vi "Version_4.9_8_on-chip_valves_for25ulSyringe_withModfied_Plunging.vi"() -> ()   [LabVIEW 2020]
uses:
  C:/Users/Admin/Desktop/MicroPurification/Developer/MainLabViewProject_V2.0/Thorlabs/Thorlabs.MotionControl.Controls.dll
  MainLabViewProject_V2.0/Thorlabs/Thorlabs.MotionControl.Controls.dll
  C:/Users/Admin/Desktop/MicroPurification/Developer/MainLabViewProject_V2.0/Thorlabs/Thorlabs.MotionControl.KCube.InertialMotorCLI.dll
  MainLabViewProject_V2.0/Thorlabs/Thorlabs.MotionControl.KCube.InertialMotorCLI.dll
  <vilib>/Instr/_visa.llb/VISA Configure Serial Port (Instr).vi
  <vilib>/Waveform/WDTOps.llb/WDT Append Waveforms DBL.vi
  <vilib>/Fluigent/Fluigent SDK/sourceCode/fgt_SDK.lvlib
panel:
  in  "Set - Blotting Time":bool
  in  "Set - Blotting Angle":bool
  in  "Automated Blotting \nand Plunging":bool=TRUE
  in  "Blotting Time":dbl=1000.0
  in  "Blotting Angle":dbl=10.0
  in  "Amount of \nGrid Shift \nfor Blotting (um)":i32
  out "Ethane Temperature":dbl
  out "RH (%)":dbl
  out "Valve Closing \nPressure Measured":sgl
  out "Suction pressure \nmeasured":sgl
  in  "Divert Elution Buffer\ninto Column-1":bool
  in  "Discard volume \npriot to elution":dbl=1.0
  in  "Buffer-B Dispense\nFlow Rate for Elution \ntubing pre-wash":dbl=2.0
  in  "Buffer-B Volume \nfor elution tubing \npre-wash":dbl=20.0
  in  "External Valve \nOpen":bool
  in  "N-B1":i32=4
  in  "Valve V10 Open":bool=TRUE
  in  "Valve V9 Open":bool=TRUE
  in  "Valve V8 Open":bool=TRUE
  in  "Capillary purge \nvolume after every\ngrid plunging":dbl=0.05
  in  "Automatic purging \nof capillary after \ngrid deposition":bool=TRUE
  in  "No. of \ncleaning cycles":i32=4
  in  "Pause Elution\nValue":dbl
  in  "Re-SEC":bool
  in  "Buffer-C2 Dispense \nFlow Rate for Washing \nPrior to re-introducing Sample":dbl=2.0
  in  "Buffer-C2 \nWash Volume\nPrior to re-introducing \nSample":dbl=20.0
  in  "Wash column-2 Prior \nto re-introducing \nsample":bool=TRUE
  in  "Valve V7 Open":bool=TRUE
  in  "Valve V6 Open":bool=TRUE
  in  "Valve V5 Open":bool=TRUE
  in  "Fluigent\nLink S/N":u16=10704
  in  "Move Grid \nDown Faster":dbl
  in  "Move Grid \nUp Faster":dbl
  in  "Affinity Elution \nGraph Min CutOff":dbl=1.0
  out "Affinity Elution \nis Approaching":bool
  out "Elution of Column-2":bool
  in  "Port for \nC2-Elution":string="5"
  out "Elution of Column-1":bool
  in  "Port for \nB-Elution":string="7"
  in  "f":dbl
  out "Washing Column-2":bool
  out "Washing Column-1":bool
  in  "Port for \nA2-Wash":string="4"
  out "Sample pumping \ninto Column-1":bool
  out "Equilibriating \nColumn-2":bool
  out "Equilibriating \nColumn-1":bool
  in  "V-S":dbl=10.0
  in  "Port for \nSample":string="3"
  in  "N-S":i32=1
  in  "External Valve \nCLOSED":string="2"
  in  "External Valve \nOPEN":string="1"
  in  "Port for \nC1-Equilibriation":string="5"
  in  "Port for \nA1-Equilibriation":string="4"
  in  "Port-<n> to be \nCleaned (4-9)":i32(ring) items=["4", "5", "6", "7", "8", "9"]
  in  "Clean the \nBuffer-C2 tubing":bool
  in  "Clean the \nBuffer-B tubing":bool=TRUE
  in  "Signal":bool
  out "Net Elution \nVolume":dbl
  out "Pause Elution":bool
  in  "Apparent Volume\nof Syringe":dbl=20.0
  in  "N-C1":i32=4
  in  "N-A1":i32=4
  in  "On-Chip Valve \nClosing\nPressure (mbar)":dbl=1200.0
  in  "Wait time for\ntranslation":u32=100
  out "Suction pressure \nfor grid deposition":sgl
  in  "Suction Pressure\nfor EM-grid \nDeposition (mbar)":sgl
  out "Amplified Signal with Fluid Volume for Affinity Elution":cluster{"Array":dbl[], "Array":dbl[]}(graph)
  out "Affinity Elution On":bool
  out "Amplified Signal with Fluid Volume Near Affinity Elution":cluster{"Array":dbl[], "Array":dbl[]}(graph)
  in  "Valve V4 Open":bool=TRUE
  out "Affinity On":bool
  out "Amplified Signal with Fluid Volume for SEC":cluster{"Array":dbl[], "Array":dbl[]}(graph)
  out "SEC On":bool
  in  "n":i32
  in  "c":dbl
  in  "Duration for \nup/down\nMovement of Grid":u32=100
  in  "Wait time before \nsolenoid for V2\nturns on 2":u32
  in  "Discard Volume":dbl
  out "Discard fluid \nprior to 1st \ndeposition":bool
  in  "Grid Deposition\nDuration":u32
  in  "Valve V3 Open":bool=TRUE
  in  "Valve V2 Open":bool=TRUE
  in  "Valve V1 Open":bool=TRUE
  in  "Delay before\n1st movement\nof grid":dbl
  in  "No of cycles\nof up-down\nmovement":dbl=7.0
  in  "Translation Step SIze\nwhile plunging":dbl=400.0
  in  "Move\nGrid Down":dbl
  in  "Move\nGrid Up":dbl
  in  "k2":dbl
  in  "k1":dbl
  in  "KCubeInertialMotorControl":refnum<k24>(container)
  in  "Select the Action":T1(ring)
  out "Temperature of Ethane Graph":waveform(dbl)(graph)
  in  "Position":i32
  out "True Volume being \ninjected in this\nprocess":dbl
  in  "Buffer-C Volume \nto be Pumped for\nColumn \nnon-interference":dbl
  in  "Buffer-C1 Dispense\nFlow Rate (ul/min) \nfor Equilibration\nof Column-2":dbl=2.0
  in  "Buffer-C1 Volume \nto be  Pumped \nfor Equilibration\nof Column-2":dbl=55.0
  in  "Buffer-C1 Pumping\nResolution \nfor Equilibration \nof Column-2":T2(ring)=enum."High Resolution Pumping"
  in  "Buffer-C1 PickUp \nFlow Rate (ul/min)\nfor Equilibration \nof Column-2":dbl=150.0
  in  "Buffer-A1 Dispense\nFlow Rate (ul/min) \nfor Equilibration\nof Column-1":dbl=2.0
  in  "Buffer-A1 Volume \nto be  Pumped \nfor Equilibration\nof Column-1":dbl=35.0
  in  "Buffer-A1 Pumping\nResolution \nfor Equilibration \nof Column-1":T2(ring)=enum."High Resolution Pumping"
  in  "Buffer-A1 PickUp \nFlow Rate (ul/min)\nfor Equilibration \nof Column-1":dbl=150.0
  out "Buffer-C Volume\nleft to be Pumped":dbl
  in  "Re-deposit Sample\nonto Grid":bool
  in  "Suction On/Off":bool
  out "Vol_previous":dbl
  out "Vol_now":dbl
  out "Position\nNow":dbl
  out "Sample Volume Diverted\ninto Column-2":dbl
  out "Reminder of the \nVolume to be \nPumped":dbl
  in  "Divert Buffer-C \ninto Column-2":bool=TRUE
  in  "Divert Sample \ninto Column-2":bool
  in  "Buffer-B Volume \nto be Pumped for\nSample Diversion\nto Column-2":dbl=0.5
  out "Amplified Signal with Fluid Volume":cluster{"Array":dbl[], "Array":dbl[]}(graph)
  in  "Stop for End of \nExperiment \nand Data Writing":bool
  in  "Select a Process":T3(ring)
  out "Initial Plunger Position":dbl
  out "Stopper that ends \nthe main loops":bool
  in  "Pause /Continue":bool
  in  "Start the Process":bool
  out "Pause Data Collection":bool
  out "Volume being Injected \ntill the end of previous \nprocess":dbl
  out "Total Volume \nbeing Injected":dbl
  out "Volume being Injected \nin this process":dbl
  in  "Divert Sample \nonto Grid":bool=TRUE
  in  "VISA Refnum in\nfor Valve":refnum<visa-resource-name>="COM3"
  in  "Buffer-C2 Dispense\nFlow Rate (ul/min)":dbl=0.25
  in  "Buffer-C2 Volume \nto be Pumped":dbl
  in  "Buffer-C2 Pumping\nResolution":T2(ring)=enum."High Resolution Pumping"
  in  "Buffer-C2 PickUp \nFlow Rate (ul/min)":dbl=150.0
  in  "Buffer-B Dispense\nFlow Rate (ul/min)":dbl=0.25
  in  "Buffer-B Volume \nto be  Pumped":dbl
  in  "Buffer-B Pumping\nResolution":T2(ring)=enum."High Resolution Pumping"
  in  "Buffer-B PickUp \nFlow Rate (ul/min)":dbl=150.0
  in  "Sample Dispense\nFlow Rate (ul/min)":dbl=2.0
  in  "Sample Volume \nto be Pumped":dbl
  in  "Sample Pumping\nResolution":T2(ring)=enum."High Resolution Pumping"
  in  "Sample PickUp \nFlow Rate (ul/min)":dbl=15.0
  in  "Buffer-A2 Dispense\nFlow Rate (ul/min)":dbl=2.0
  in  "Buffer-A2 Volume \nto be Pumped":dbl
  in  "Buffer-A2 Pumping\nResolution":T2(ring)=enum."High Resolution Pumping"
  in  "Buffer-A2 PickUp \nFlow Rate (ul/min)":dbl=150.0
  in  "Volume of Syringe":dbl=25.0
  in  "VISA Refnum in\nfor Pump":refnum<visa-resource-name>="COM4"
  # "More Notes:\n\n- At the start of the experiment, ensure the extrenal valve is detected by teh program\\\n            - Manually unplug and replug the power connection to the valve (locatd near the valve)\n            - Start the program and click on 'Initialize only the valve\" and click on \"Start the Process\"\n            \n\n              - If the program doesn't initialize the valve in 30 sec, turn off the program.\n             -  Manually unplug and replug the power connection to the valve (locatd near the valve) again\n             - Start the LSPone quick softwar on teh desktop and click on the Mnual setting\n             - Choose 'COM3'\n             - Click on Initialize. If teh initialization is sucessful, close this isftware and turn on the \n                 Labview program and try to inialize teh valve. If the valve gets initialized, you are \n                  good to go and use the program further, else redo the process.\n\n- After the above step, while cleaning the tubings\n             - First cleaning ttubings using IPA ....The code is 'clean tubings 3,4, 5and 7\n             - Clean the tubing that goes to teh chip affinity column twice using IPA, run Buffer-A2 pumping code\n             - Clean the tubing that goes to teh chip SEC column twice using IPA, run Buffer-C2 pumping code\n              - Run the above 3 steps with IPA again. This ensures we have teh least bubbles in teh sysetm\n              - Run the 1st 3 steps with water.\n              - After inserting the tubings to the chip, clean teh affinity and SEC columns at 2 ul/min of 30 ul each with water\n              - Before teh start of the main experimnet, run the  code 'clean the tubing from port-3 vial' with Buffer-A once\n\n               - Place teh sample and all teh buffers in the appropriate places and run teh code  with Re-SEC possibility with \n                  appropriate parameters"
  # "Clean only 3,4,5 and 7 \nfor Complex-I\nunless other ports are used"
  # "Notes specific for this code:\n\n- V1 is teh valve just prior to and after affinity column, all other valves are numbered \nclockwise with valve V8 to be teh valve conncecting affinity inlet to waste outlet-2.\n\n- V9 and V10 are valves for affinity wash and elution inlets. Currently they are not used \nin this code.\n\n- Port-8 is connected to the tubing of elution that is conncetcted to column-1 of chip"
  # "Pump Port No           Function\n         1                       Pump Waste\n         2                       Chip Column-1 Connection\n         3                       Sample\n         4                       Buffer- A1 for Equilibriation of Column-1\n         5                       Buffer- C1 for Equilibriation of Column-2\n         6                       Buffer- A2 for Wash of Column-1\n         7                       Buffer- B for Elution of Column-1\n         8                       Buffer-C2 for Elution of Column-2\n         9                       Buffer- A3 for Wash of Column-1\n        10                      Chip Column-2 Connection"
  # "Column-2 Wash Parameters"
  # "Notes:\n- This code uses USB6002 data acquisition device from NI\n- No PGA and only AD8611ARZ preamp\n- Still uses Arduino Uno and Stepper motor \n- Even though designed for Complex-I, but is more generic\n- The code is meant for a chip with 7-onchip valves that are being \ncontrolled using fluigent P-switch, one external on/off valve\nand the pump with 10 ports\n- The tubings \n            - 0.18 mm ID tubings from port-2 to chip, port-3 to sample vial, \nport-10 to SEC inlet of the chip, port-1 to pump-waste\n             - 0.5 mm ID tubings from port-4 to Buffer-A vial, port-5 to \nBuffer-C vial, and port-7 to Buffer-B vial"
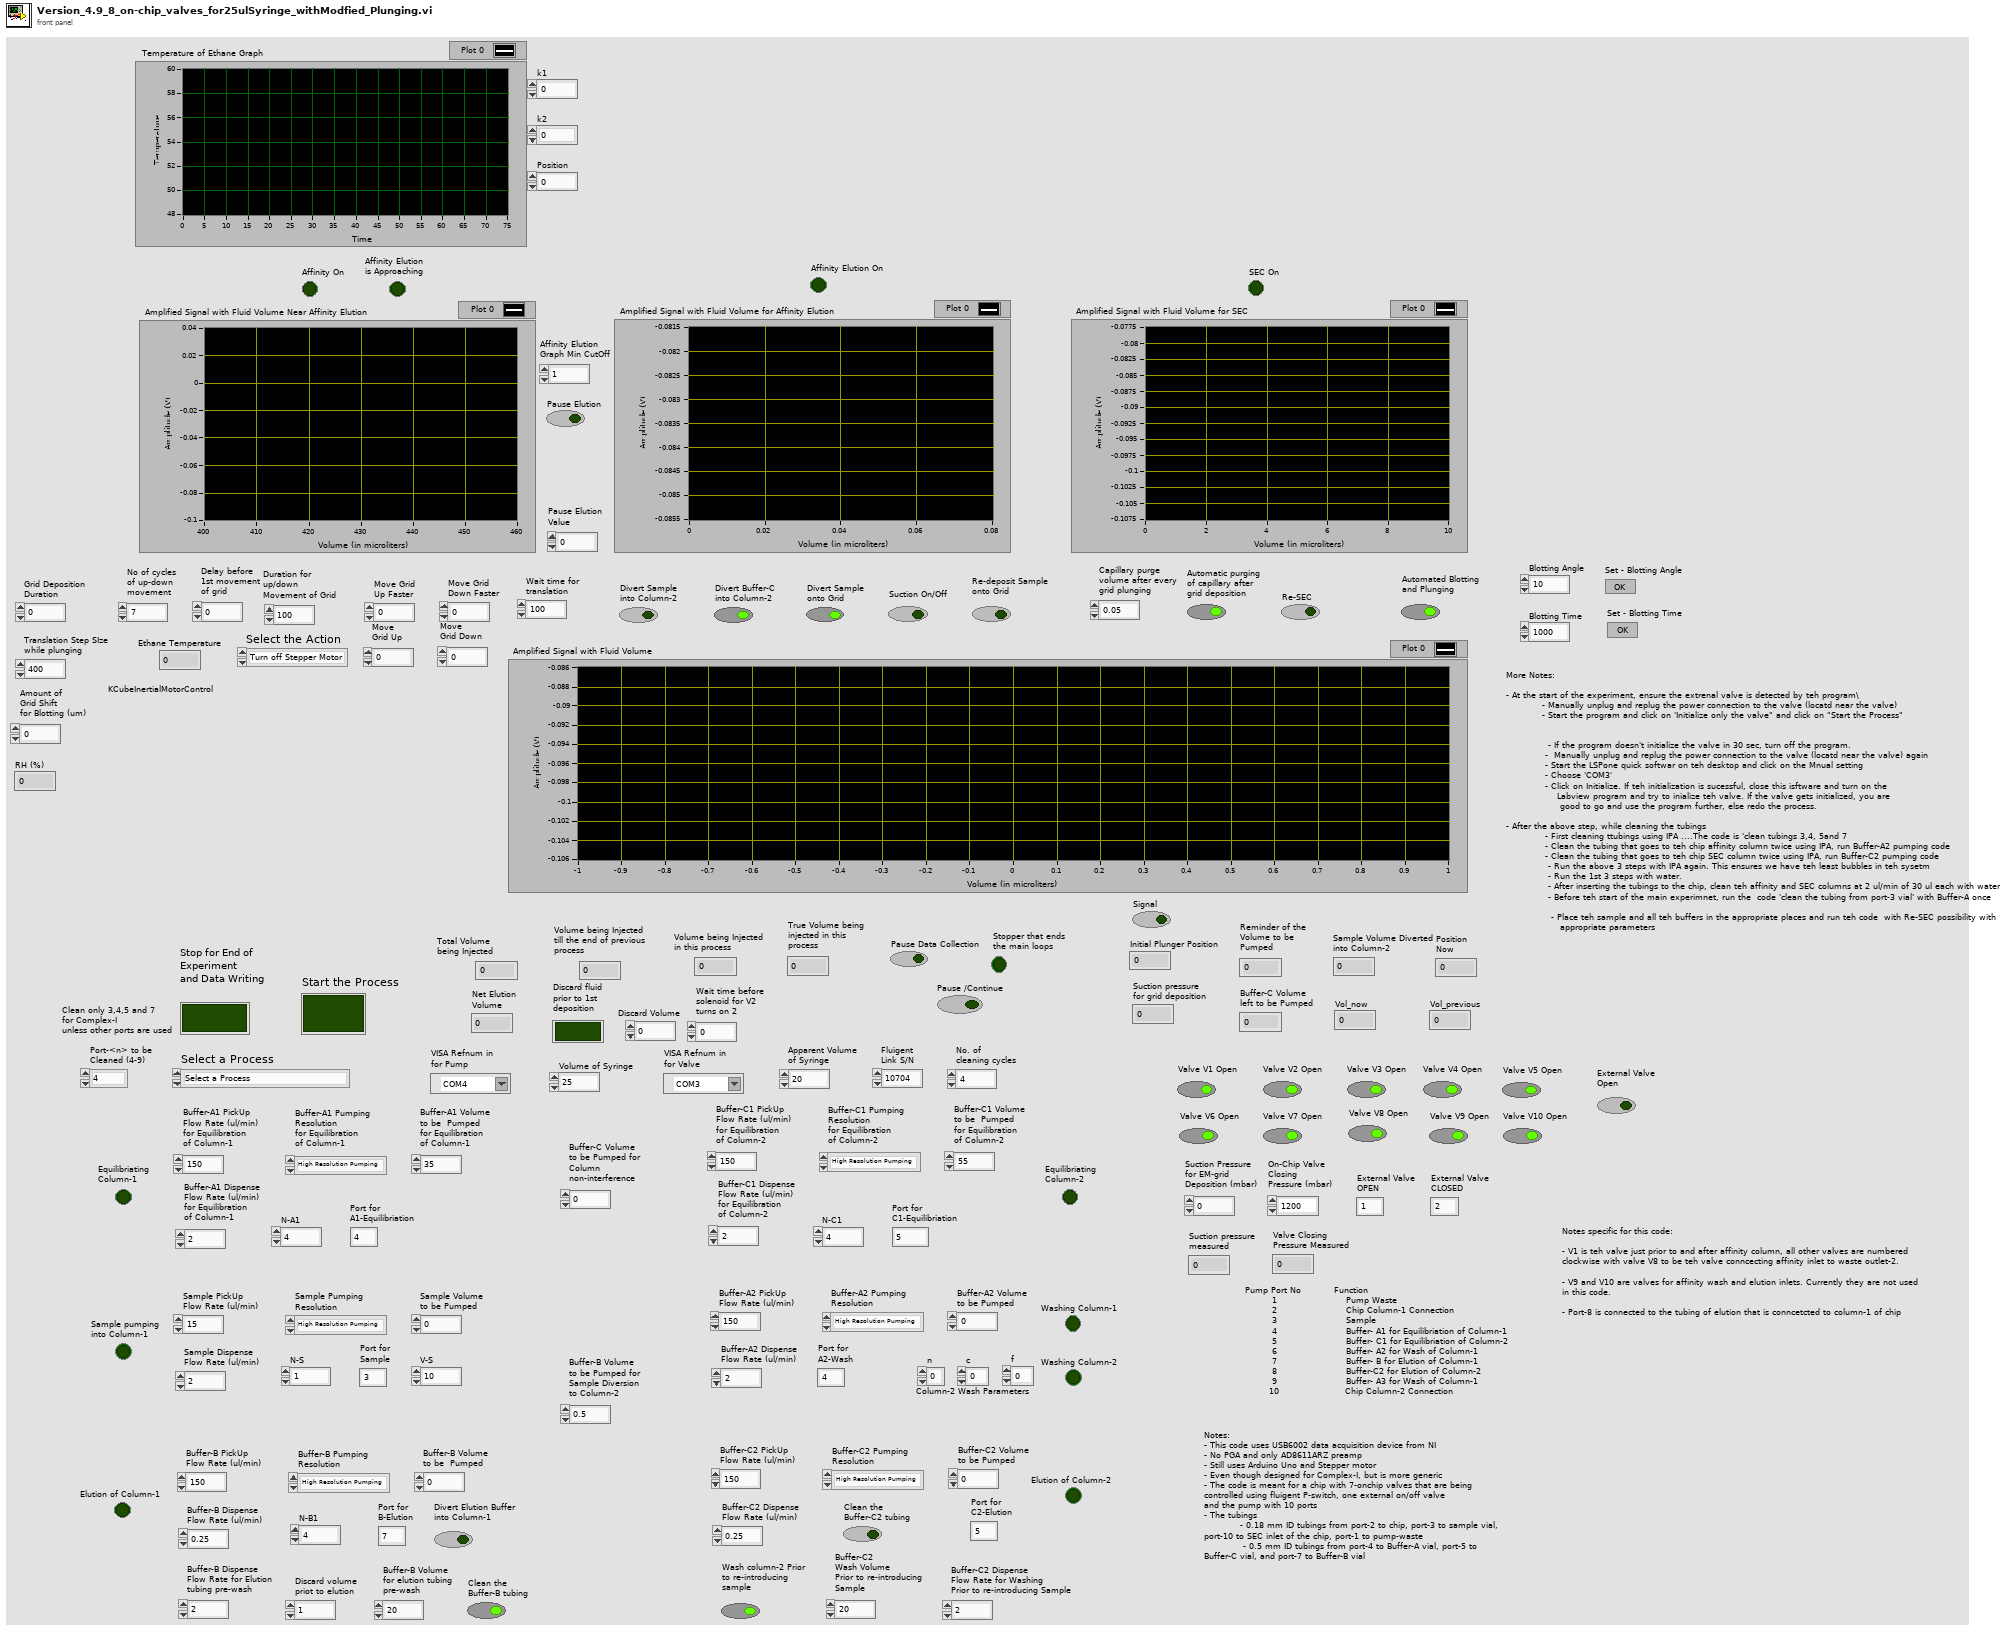
[diagram p1: front panel]
types:
  T1 = enum16{"Turn off Stepper Motor", "Turn  on Stepper Motor", "Spread the deposited protein on the grid in One Line and plunge", "Spread the deposited protein on the grid and plunge", "Start Plunging", "Reset Plunger"}
  T2 = enum16{"Standard Pumping", "High Resolution Pumping"}
  T3 = enum16{"Select a Process", "Initialize Only The Pump", "Initialize Only the Valve", "Initialize Pump and Valve", "Clean the tubing from Port-3 Vial", "Clean the tubing from Port-<n> Vial", "Clean the tubing from Ports 3,4,5 and 7", "Automated Protein Purification with Re-SEC Possibility, 8 SOD Valves and On/Off External Valve", "Automated Protein Purification with 7 SOD Valves and On/Off External Valve", "Automated Plunging Alone Using Purified Protein Via Chip", "Automated Plunging alone using purified protein from SEC column", "Inject Buffer A2, Column 1 with 4 SOD Valves", "Inject Sample, Column 1", "Inject Buffer B, Column 1 with 4 SOD Valves", "Inject Buffer C2, Column 2 with 4 SOD Valves", "Check_Suction_Valve_functionality"}
diagram:
  # "Valve V3 is the on-chip SOD Valve that is after the column-2, after valve V1 and on the way to the waste outlet"
  # "Valve V2 is the on-chip SOD Valve that is after the column-2, after valve V1 and on the way to capillary."
  # "Valve V1 is the on-chip SOD Valve that is after the column-2, just after detection zone-2"
  # "Valve V4 is the on-chip SOD Valve that is after the column-1, just prior to column-2"
  n1 = stacked-sequence {
    frame #0 {
      # "Plunger Control and Ethane Chamber Temperature Display"
      # "AMPLIFIER BLOCK"
      n2 = property class="KCubeInertialMotorControl"(reference="KCubeInertialMotorControl", "SerialNumber"="97102163" ("Serial Number")) -> (reference out=w74:refnum<k24>, error out=w81:errorcluster)  [unwired: 1 in]
      n3 = while {
        stop <- w525 stop-if-true
        n4 = case shown="\"Automated Protein Purification with Re-SEC Possibility, 8 SOD Valves and On/Off External Valve\"" "Select a Process" {
          frame "Initialize Pump and Valve" {
            n5 = local read "Stop for End of \nExperiment \nand Data Writing"() -> (w527:bool)
            n6 = case shown="False" w527 {
              frame False {
                n7 = local read "Start the Process"() -> (w528:bool)
                n8 = case shown="True" w528 {
                  frame False {
                    n9 = local read "Stopper that ends \nthe main loops"() -> (w530:bool)
                    n10 = local read "Start the Process"() -> (w531:bool)
                    n11 = Or(x=w531, y=w530) -> (x .or. y?=w529:bool)
                    n12 = case shown="False" w529 {
                      frame False {
                        n13 = while {
                          stop <- w534 stop-if-true
                          n14 = local read "Stopper that ends \nthe main loops"() -> (w536:bool)
                          n15 = local read "Start the Process"() -> (w535:bool)
                          n16 = Or(x=w535, y=w536) -> (x .or. y?=w534:bool)
                          n17 = Wait (ms)(milliseconds to wait=u32 10) -> ()  [unwired: 1 out]
                        }
                        n18 = One Button Dialog(message="Please select the process and press the 'Start Process' Button") -> ()  [unwired: 1 in, 1 out]
                      }
                      frame True {
                      }
                    }
                  }
                  frame True {
                    n19 = stacked-sequence {
                      frame #0 {
                        n20 = local read "VISA Refnum in\nfor Pump"() -> (w537:refnum<visa-resource-name>)
                        n21 = call "Initializer (SubVI).vi"("VISA Refnum in"=w537) -> ()  [unwired: 11 in]
                      }
                      frame #1 {
                        n22 = local read "VISA Refnum in\nfor Pump"() -> (w538:refnum<visa-resource-name>)
                        n23 = call "ProcessCompletionWaiter (SubVI).vi"("VISA Refnum in"=w538) -> ()  [unwired: 11 in]
                      }
                      frame #2 {
                        n24 = local read "VISA Refnum in\nfor Valve"() -> (w539:refnum<visa-resource-name>)
                        n25 = call "Initializer_Valve (SubVI).vi"("VISA Refnum in"=w539) -> ()  [unwired: 11 in]
                      }
                      frame #3 {
                        n26 = local read "VISA Refnum in\nfor Valve"() -> (w540:refnum<visa-resource-name>)
                        n27 = call "ProcessCompletionWaiter (SubVI).vi"("VISA Refnum in"=w540) -> ()  [unwired: 11 in]
                      }
                      frame #4 {
                        n28 = local write "Start the Process"(FALSE ("Start the Process")) -> ()
                      }
                    }
                  }
                }
              }
              frame True {
              }
            }
          }
          frame "Inject Sample, Column 1" {
            n29 = local read "Stopper that ends \nthe main loops"() -> (w542:bool)
            n30 = case shown="False" w542 {
              frame False {
                n31 = local read "Start the Process"() -> (w543:bool)
                n32 = case shown="True" w543 {
                  frame False {
                    n33 = local read "Stopper that ends \nthe main loops"() -> (w545:bool)
                    n34 = local read "Start the Process"() -> (w544:bool)
                    n35 = Or(x=w545, y=w544) -> (x .or. y?=w546:bool)
                    n36 = case shown="False" w546 {
                      frame False {
                        n37 = while {
                          stop <- w549 stop-if-true
                          n38 = local read "Stopper that ends \nthe main loops"() -> (w551:bool)
                          n39 = local read "Stop for End of \nExperiment \nand Data Writing"() -> (w548:bool)
                          n40 = local read "Start the Process"() -> (w550:bool)
                          n41 = Wait (ms)(milliseconds to wait=u32 10) -> ()  [unwired: 1 out]
                          n42 = Or(x=w551, y=w550) -> (x .or. y?=w549:bool)
                          n43 = local write "Stopper that ends \nthe main loops"(w548) -> ()
                        }
                        n44 = One Button Dialog(message="Please Select the Process and Press 'Start the Process' Button") -> ()  [unwired: 1 in, 1 out]
                      }
                      frame True {
                      }
                    }
                  }
                  frame True {
                    n45 = stacked-sequence {
                      frame #0 {
                        n46 = local read "Sample Volume \nto be Pumped"() -> (w556:dbl)
                        n47 = local read "Apparent Volume\nof Syringe"() -> (w555:dbl)
                        n48 = Quotient & Remainder(x=w556, y=w555) -> (x-y*floor(x/y)=w554:dbl, floor(x/y)=w553:dbl)
                        n49 = for {
                          N: w553 -> [_]
                          n50 = stacked-sequence {
                            frame #0 {
                              # "Switch to Port-3"
                              # "Port-3 of pump is connected to Sample"
                              n51 = local read "VISA Refnum in\nfor Pump"() -> (w558:refnum<visa-resource-name>)
                              n52 = local read "Port for \nSample"() -> (w557:string)
                              n53 = call "PortChanger (SubVI).vi"("Port Number"=w557, "VISA Refnum in"=w558) -> ()  [unwired: 10 in]
                            }
                            frame #1 {
                              n54 = local read "VISA Refnum in\nfor Pump"() -> (w559:refnum<visa-resource-name>)
                              n55 = call "ProcessCompletionWaiter (SubVI).vi"("VISA Refnum in"=w559) -> ()  [unwired: 11 in]
                            }
                            frame #2 {
                              n56 = local read "Sample PickUp \nFlow Rate (ul/min)"() -> (w562:dbl)
                              n57 = local read "Sample Pumping\nResolution"() -> (w561:T2)
                              n58 = local read "VISA Refnum in\nfor Pump"() -> (w564:refnum<visa-resource-name>)
                              n59 = local read "Apparent Volume\nof Syringe"() -> (w560:dbl)
                              n60 = local read "Volume of Syringe"() -> (w563:dbl)
                              n61 = call "RPickUp(SubVI).vi"("Volume to be picked up"=w560, "Volume of Syringe"=w563, "Resolution of PickUP"=w561, "PickUp Flow Rate (ul/min)"=w562, "VISA Refnum in"=w564) -> ()  [unwired: 6 in, 1 out]
                            }
                            frame #3 {
                              n62 = local read "Stopper that ends \nthe main loops"() -> (w565:bool)
                              n63 = local read "VISA Refnum in\nfor Pump"() -> (w566:refnum<visa-resource-name>)
                              n64 = case shown="True" w565 {
                                frame False {
                                }
                                frame True {
                                n65 = local read "VISA Refnum in\nfor Pump"() -> (w567:refnum<visa-resource-name>)
                                n66 = call "HardStopCurrentProcess (SubVI).vi"("VISA Refnum in"=w567) -> ()  [unwired: 11 in]
                                }
                              }
                              n67 = call "ProcessCompletionWaiter (SubVI).vi"("VISA Refnum in"=w566) -> ()  [unwired: 11 in]
                            }
                            frame #4 {
                              # "Reads the initial Plunger Position for computing the volume dispensed"
                              n68 = local read "VISA Refnum in\nfor Pump"() -> (w569:refnum<visa-resource-name>)
                              n69 = call "AbsolutePlungerPosition (SubVI).vi"("VISA Refnum in"=w569) -> ("Plunger Position"=w568:i32)  [unwired: 10 in]
                              n70 = local write "Initial Plunger Position"(w568) -> ()
                            }
                            frame #5 {
                              # "Switch to Port-2"
                              # "Port-2 of the pump is conncted to column-1 of chip"
                              n71 = local read "VISA Refnum in\nfor Pump"() -> (w571:refnum<visa-resource-name>)
                              n72 = call "PortChanger (SubVI).vi"("Port Number"="2", "VISA Refnum in"=w571) -> ()  [unwired: 10 in]
                            }
                            frame #6 {
                              n73 = local read "Stopper that ends \nthe main loops"() -> (w572:bool)
                              n74 = local read "VISA Refnum in\nfor Pump"() -> (w573:refnum<visa-resource-name>)
                              n75 = case shown="True" w572 {
                                frame False {
                                }
                                frame True {
                                n76 = local read "VISA Refnum in\nfor Pump"() -> (w574:refnum<visa-resource-name>)
                                n77 = call "HardStopCurrentProcess (SubVI).vi"("VISA Refnum in"=w574) -> ()  [unwired: 11 in]
                                }
                              }
                              n78 = call "ProcessCompletionWaiter (SubVI).vi"("VISA Refnum in"=w573) -> ()  [unwired: 11 in]
                            }
                            frame #7 {
                              # "Keeps the AMF valve after column-1 open and valve after column-2 closed"
                              n79 = local read "Sample Dispense\nFlow Rate (ul/min)"() -> (w587:dbl)
                              n80 = local read "Sample Pumping\nResolution"() -> (w586:T2)
                              n81 = local read "VISA Refnum in\nfor Pump"() -> (w589:refnum<visa-resource-name>)
                              n82 = local write "Pause Data Collection"(FALSE ("Pause Data Collection")) -> ()
                              n83 = local read "Volume of Syringe"() -> (w588:dbl)
                              n84 = call "GoToAbsolutePosition(SubVI).vi"("Absolute Volume Position in Syringe (in ul)"=0.0 ("Volume to be Dispensed"), "Volume of Syringe"=w588, "Resolution of Pumping"=w586, "Flow Rate (ul/min)"=w587, "VISA Refnum in"=w589) -> ()  [unwired: 6 in, 1 out]
                              n85 = local write "Valve V1 Open"(TRUE ("Valve V1 Open")) -> ()
                              n86 = local write "Valve V2 Open"(TRUE ("Valve V2 Open")) -> ()
                              n87 = local write "Valve V3 Open"(FALSE ("Valve V3 Open")) -> ()
                              n88 = local write "Valve V4 Open"(FALSE ("Valve V4 Open")) -> ()
                              n89 = local write "External Valve \nOpen"(TRUE ("External Valve \nOpen")) -> ()
                              n90 = local write "Valve V8 Open"(FALSE ("Valve V8 Open")) -> ()
                              n91 = local write "Valve V5 Open"(FALSE ("Valve V5 Open")) -> ()
                              n92 = local write "Valve V6 Open"(FALSE ("Valve V6 Open")) -> ()
                              n93 = local write "Valve V7 Open"(FALSE ("Valve V7 Open")) -> ()
                            }
                            frame #8 {
                              n94 = local read "Initial Plunger Position"() -> (w592:dbl)
                              n95 = local read "Sample Pumping\nResolution"() -> (w591:T2)
                              n96 = local read "VISA Refnum in\nfor Pump"() -> (w593:refnum<visa-resource-name>)
                              n97 = local read "Volume of Syringe"() -> (w590:dbl)
                              n98 = stacked-sequence {
                                tunnel: w590 -> [w594]
                                tunnel: w591 -> [w595]
                                tunnel: w592 -> [w597]
                                tunnel: w593 -> [w596]
                                frame #0 {
                                n99 = while {
                                tunnel: w597 -> [w603]
                                tunnel: w596 -> [w602]
                                tunnel: w595 -> [w601]
                                tunnel: w594 -> [w600]
                                stop <- w598 stop-if-true
                                n100 = Wait (ms)(milliseconds to wait=u32 100) -> ()  [unwired: 1 out]
                                n101 = stacked-sequence {
                                tunnel: w603 -> [w609 _]
                                tunnel: w602 -> [w608 w629]
                                tunnel: w601 -> [w607 _]
                                tunnel: w600 -> [w606 _]
                                tunnel: [_ w626] -> w598
                                frame #0 {
                                n102 = call "AbsolutePlungerPosition (SubVI).vi"("VISA Refnum in"=w608) -> ("Plunger Position"=w605:i32)  [unwired: 10 in]
                                n103 = case shown="\"Standard Pumping\", Default" w607 {
                                tunnel: w609 -> [w614 w623]
                                tunnel: w605 -> [w615 w622]
                                tunnel: [w613 w620] -> w604
                                tunnel: w606 -> [w612 w621]
                                frame "Standard Pumping", Default {
                                n104 = Subtract(x=w614, y=w615) -> (x-y=w611:dbl)
                                n105 = Absolute Value(x=w611) -> (abs(x)=w610:dbl)
                                n106 = Multiply(x=w610, y=w612) -> (x*y=w617:dbl)
                                n107 = Divide(x=w617, y=3000.0) -> (x/y=w613:dbl)
                                }
                                frame "High Resolution Pumping" {
                                n108 = Subtract(x=w623, y=w622) -> (x-y=w619:dbl)
                                n109 = Absolute Value(x=w619) -> (abs(x)=w618:dbl)
                                n110 = Multiply(x=w618, y=w621) -> (x*y=w625:dbl)
                                n111 = Divide(x=w625, y=24000.0) -> (x/y=w620:dbl)
                                }
                                }
                                n112 = local write "Volume being Injected \nin this process"(w604) -> ()
                                }
                                frame #1 {
                                n113 = local read "Stopper that ends \nthe main loops"() -> (w628:bool)
                                n114 = call "LSPOneStatus (SubVI).vi"("VISA Refnum in"=w629) -> ("read buffer"=w631:string)  [unwired: 10 in]
                                n115 = call <vilib>:"Trim Whitespace.vi"("string"=w631) -> ("trimmed string"=w630:string)  [unwired: 1 in]
                                n116 = Equal?(x=w630, y="/0`\u0003") -> (x = y?=w627:bool)
                                n117 = Or(x=w627, y=w628) -> (x .or. y?=w626:bool)
                                }
                                }
                                }
                                }
                              }
                            }
                            frame #9 {
                              n118 = local read "Stopper that ends \nthe main loops"() -> (w633:bool)
                              n119 = local write "Pause Data Collection"(TRUE ("Pause Data Collection")) -> ()
                              n120 = local write "Valve V1 Open"(FALSE ("Valve V1 Open")) -> ()
                              n121 = local write "Valve V2 Open"(FALSE ("Valve V2 Open")) -> ()
                              n122 = local write "Valve V3 Open"(FALSE ("Valve V3 Open")) -> ()
                              n123 = local write "Valve V4 Open"(FALSE ("Valve V4 Open")) -> ()
                              n124 = Wait (ms)(milliseconds to wait=u32 500) -> ()  [unwired: 1 out]
                              n125 = case shown="True" w633 {
                                frame False {
                                }
                                frame True {
                                n126 = local read "VISA Refnum in\nfor Pump"() -> (w643:refnum<visa-resource-name>)
                                n127 = call "HardStopCurrentProcess (SubVI).vi"("VISA Refnum in"=w643) -> ()  [unwired: 11 in]
                                }
                              }
                              n128 = local write "Valve V5 Open"(FALSE ("Valve V5 Open")) -> ()
                              n129 = local write "Valve V6 Open"(FALSE ("Valve V6 Open")) -> ()
                              n130 = local write "Valve V7 Open"(FALSE ("Valve V7 Open")) -> ()
                            }
                            frame #10 {
                              n131 = local write "Volume being Injected \nin this process"(0.0 ("Volume being Injected \nin this process")) -> ()
                            }
                          }
                        }
                        n132 = local write "Reminder of the \nVolume to be \nPumped"(w554) -> ()
                      }
                      frame #1 {
                        n133 = stacked-sequence {
                          frame #0 {
                            # "Switch to Port-3"
                            # "Port-3 of pump is connected to Sample"
                            n134 = local read "VISA Refnum in\nfor Pump"() -> (w646:refnum<visa-resource-name>)
                            n135 = local read "Port for \nSample"() -> (w645:string)
                            n136 = call "PortChanger (SubVI).vi"("Port Number"=w645, "VISA Refnum in"=w646) -> ()  [unwired: 10 in]
                          }
                          frame #1 {
                            n137 = local read "VISA Refnum in\nfor Pump"() -> (w647:refnum<visa-resource-name>)
                            n138 = call "ProcessCompletionWaiter (SubVI).vi"("VISA Refnum in"=w647) -> ()  [unwired: 11 in]
                          }
                          frame #2 {
                            n139 = local read "Sample PickUp \nFlow Rate (ul/min)"() -> (w650:dbl)
                            n140 = local read "Sample Pumping\nResolution"() -> (w649:T2)
                            n141 = local read "VISA Refnum in\nfor Pump"() -> (w652:refnum<visa-resource-name>)
                            n142 = local read "Reminder of the \nVolume to be \nPumped"() -> (w648:dbl)
                            n143 = local read "Volume of Syringe"() -> (w651:dbl)
                            n144 = call "RPickUp(SubVI).vi"("Volume to be picked up"=w648, "Volume of Syringe"=w651, "Resolution of PickUP"=w649, "PickUp Flow Rate (ul/min)"=w650, "VISA Refnum in"=w652) -> ()  [unwired: 6 in, 1 out]
                          }
                          frame #3 {
                            n145 = local read "Stopper that ends \nthe main loops"() -> (w653:bool)
                            n146 = local read "VISA Refnum in\nfor Pump"() -> (w654:refnum<visa-resource-name>)
                            n147 = case shown="True" w653 {
                              frame False {
                              }
                              frame True {
                                n148 = local read "VISA Refnum in\nfor Pump"() -> (w655:refnum<visa-resource-name>)
                                n149 = call "HardStopCurrentProcess (SubVI).vi"("VISA Refnum in"=w655) -> ()  [unwired: 11 in]
                              }
                            }
                            n150 = call "ProcessCompletionWaiter (SubVI).vi"("VISA Refnum in"=w654) -> ()  [unwired: 11 in]
                          }
                          frame #4 {
                            # "Reads the initial Plunger Position for computing the volume dispensed"
                            n151 = local read "VISA Refnum in\nfor Pump"() -> (w657:refnum<visa-resource-name>)
                            n152 = call "AbsolutePlungerPosition (SubVI).vi"("VISA Refnum in"=w657) -> ("Plunger Position"=w656:i32)  [unwired: 10 in]
                            n153 = local write "Initial Plunger Position"(w656) -> ()
                          }
                          frame #5 {
                            # "Switch to Port-2"
                            # "Port-2 of the pump is conncted to column-1 of chip"
                            n154 = local read "VISA Refnum in\nfor Pump"() -> (w659:refnum<visa-resource-name>)
                            n155 = call "PortChanger (SubVI).vi"("Port Number"="2", "VISA Refnum in"=w659) -> ()  [unwired: 10 in]
                          }
                          frame #6 {
                            n156 = local read "Stopper that ends \nthe main loops"() -> (w660:bool)
                            n157 = local read "VISA Refnum in\nfor Pump"() -> (w661:refnum<visa-resource-name>)
                            n158 = case shown="True" w660 {
                              frame False {
                              }
                              frame True {
                                n159 = local read "VISA Refnum in\nfor Pump"() -> (w662:refnum<visa-resource-name>)
                                n160 = call "HardStopCurrentProcess (SubVI).vi"("VISA Refnum in"=w662) -> ()  [unwired: 11 in]
                              }
                            }
                            n161 = call "ProcessCompletionWaiter (SubVI).vi"("VISA Refnum in"=w661) -> ()  [unwired: 11 in]
                          }
                          frame #7 {
                            # "Keeps the AMF valve after column-1 open and valve after column-2 closed"
                            n162 = local read "Sample Dispense\nFlow Rate (ul/min)"() -> (w675:dbl)
                            n163 = local read "Sample Pumping\nResolution"() -> (w674:T2)
                            n164 = local read "VISA Refnum in\nfor Pump"() -> (w677:refnum<visa-resource-name>)
                            n165 = local write "Pause Data Collection"(FALSE ("Pause Data Collection")) -> ()
                            n166 = local read "Volume of Syringe"() -> (w676:dbl)
                            n167 = call "GoToAbsolutePosition(SubVI).vi"("Absolute Volume Position in Syringe (in ul)"=0.0 ("Volume to be Dispensed"), "Volume of Syringe"=w676, "Resolution of Pumping"=w674, "Flow Rate (ul/min)"=w675, "VISA Refnum in"=w677) -> ()  [unwired: 6 in, 1 out]
                            n168 = local write "Valve V1 Open"(TRUE ("Valve V1 Open")) -> ()
                            n169 = local write "Valve V2 Open"(TRUE ("Valve V2 Open")) -> ()
                            n170 = local write "Valve V3 Open"(FALSE ("Valve V3 Open")) -> ()
                            n171 = local write "Valve V4 Open"(FALSE ("Valve V4 Open")) -> ()
                            n172 = local write "External Valve \nOpen"(TRUE ("External Valve \nOpen")) -> ()
                            n173 = local write "Valve V5 Open"(FALSE ("Valve V5 Open")) -> ()
                            n174 = local write "Valve V6 Open"(FALSE ("Valve V6 Open")) -> ()
                            n175 = local write "Valve V7 Open"(FALSE ("Valve V7 Open")) -> ()
                            n176 = local write "Valve V8 Open"(FALSE ("Valve V8 Open")) -> ()
                          }
                          frame #8 {
                            n177 = local read "Initial Plunger Position"() -> (w680:dbl)
                            n178 = local read "Sample Pumping\nResolution"() -> (w679:T2)
                            n179 = local read "VISA Refnum in\nfor Pump"() -> (w681:refnum<visa-resource-name>)
                            n180 = local read "Volume of Syringe"() -> (w678:dbl)
                            n181 = stacked-sequence {
                              tunnel: w678 -> [w682]
                              tunnel: w679 -> [w683]
                              tunnel: w680 -> [w685]
                              tunnel: w681 -> [w684]
                              frame #0 {
                                n182 = while {
                                tunnel: w685 -> [w691]
                                tunnel: w684 -> [w690]
                                tunnel: w683 -> [w689]
                                tunnel: w682 -> [w688]
                                stop <- w686 stop-if-true
                                n183 = Wait (ms)(milliseconds to wait=u32 100) -> ()  [unwired: 1 out]
                                n184 = stacked-sequence {
                                tunnel: w691 -> [w697 _]
                                tunnel: w690 -> [w696 w717]
                                tunnel: w689 -> [w695 _]
                                tunnel: w688 -> [w694 _]
                                tunnel: [_ w714] -> w686
                                frame #0 {
                                n185 = call "AbsolutePlungerPosition (SubVI).vi"("VISA Refnum in"=w696) -> ("Plunger Position"=w693:i32)  [unwired: 10 in]
                                n186 = case shown="\"Standard Pumping\", Default" w695 {
                                tunnel: w697 -> [w702 w711]
                                tunnel: w693 -> [w703 w710]
                                tunnel: [w701 w708] -> w692
                                tunnel: w694 -> [w700 w709]
                                frame "Standard Pumping", Default {
                                n187 = Subtract(x=w702, y=w703) -> (x-y=w699:dbl)
                                n188 = Absolute Value(x=w699) -> (abs(x)=w698:dbl)
                                n189 = Multiply(x=w698, y=w700) -> (x*y=w705:dbl)
                                n190 = Divide(x=w705, y=3000.0) -> (x/y=w701:dbl)
                                }
                                frame "High Resolution Pumping" {
                                n191 = Subtract(x=w711, y=w710) -> (x-y=w707:dbl)
                                n192 = Absolute Value(x=w707) -> (abs(x)=w706:dbl)
                                n193 = Multiply(x=w706, y=w709) -> (x*y=w713:dbl)
                                n194 = Divide(x=w713, y=24000.0) -> (x/y=w708:dbl)
                                }
                                }
                                n195 = local write "Volume being Injected \nin this process"(w692) -> ()
                                }
                                frame #1 {
                                n196 = local read "Stopper that ends \nthe main loops"() -> (w716:bool)
                                n197 = call "LSPOneStatus (SubVI).vi"("VISA Refnum in"=w717) -> ("read buffer"=w719:string)  [unwired: 10 in]
                                n198 = call <vilib>:"Trim Whitespace.vi"("string"=w719) -> ("trimmed string"=w718:string)  [unwired: 1 in]
                                n199 = Equal?(x=w718, y="/0`\u0003") -> (x = y?=w715:bool)
                                n200 = Or(x=w715, y=w716) -> (x .or. y?=w714:bool)
                                }
                                }
                                }
                              }
                            }
                          }
                          frame #9 {
                            n201 = local read "Stopper that ends \nthe main loops"() -> (w721:bool)
                            n202 = local write "Pause Data Collection"(TRUE ("Pause Data Collection")) -> ()
                            n203 = local write "Start the Process"(FALSE) -> ()
                            n204 = local write "Valve V1 Open"(FALSE ("Valve V1 Open")) -> ()
                            n205 = local write "Valve V2 Open"(FALSE ("Valve V2 Open")) -> ()
                            n206 = local write "Valve V3 Open"(FALSE ("Valve V3 Open")) -> ()
                            n207 = local write "Valve V4 Open"(FALSE ("Valve V4 Open")) -> ()
                            n208 = Wait (ms)(milliseconds to wait=u32 500) -> ()  [unwired: 1 out]
                            n209 = case shown="True" w721 {
                              frame False {
                              }
                              frame True {
                                n210 = local read "VISA Refnum in\nfor Pump"() -> (w732:refnum<visa-resource-name>)
                                n211 = call "HardStopCurrentProcess (SubVI).vi"("VISA Refnum in"=w732) -> ()  [unwired: 11 in]
                              }
                            }
                            n212 = local write "Valve V5 Open"(FALSE ("Valve V5 Open")) -> ()
                            n213 = local write "Valve V6 Open"(FALSE ("Valve V6 Open")) -> ()
                            n214 = local write "Valve V7 Open"(FALSE ("Valve V7 Open")) -> ()
                          }
                          frame #10 {
                            n215 = local write "Volume being Injected \nin this process"(0.0 ("Volume being Injected \nin this process")) -> ()
                          }
                        }
                      }
                    }
                  }
                }
              }
              frame True {
                n216 = local write "Pause Data Collection"(FALSE ("Pause Data Collection")) -> ()
              }
            }
          }
          frame "Select a Process" {
            n217 = local read "Stopper that ends \nthe main loops"() -> (w735:bool)
            n218 = case shown="False" w735 {
              frame False {
                n219 = stacked-sequence {
                  frame #0 {
                    n220 = local write "Pause Data Collection"(TRUE ("Pause Data Collection")) -> ()
                    n221 = local write "Start the Process"(FALSE ("Start the Process")) -> ()
                  }
                  frame #1 {
                    n222 = local read "Stopper that ends \nthe main loops"() -> (w739:bool)
                    n223 = local read "Start the Process"() -> (w740:bool)
                    n224 = Or(x=w740, y=w739) -> (x .or. y?=w738:bool)
                    n225 = case shown="False" w738 {
                      frame False {
                        n226 = while {
                          stop <- w744 stop-if-true
                          n227 = local read "Stopper that ends \nthe main loops"() -> (w745:bool)
                          n228 = local read "Start the Process"() -> (w746:bool)
                          n229 = local read "Stop for End of \nExperiment \nand Data Writing"() -> (w742:bool)
                          n230 = Wait (ms)(milliseconds to wait=u32 10) -> ()  [unwired: 1 out]
                          n231 = Or(x=w746, y=w745) -> (x .or. y?=w744:bool)
                          n232 = local write "Stopper that ends \nthe main loops"(w742) -> ()
                        }
                        n233 = One Button Dialog(message="Please Select the Process and Press the 'Start the Process' Button") -> ()  [unwired: 1 in, 1 out]
                      }
                      frame True {
                      }
                    }
                  }
                }
              }
              frame True {
                n234 = local write "Pause Data Collection"(FALSE ("Pause Data Collection")) -> ()
              }
            }
          }
          frame "Clean the tubing from Port-3 Vial" {
            n235 = local read "Stopper that ends \nthe main loops"() -> (w748:bool)
            n236 = case shown="False" w748 {
              frame False {
                n237 = local read "Start the Process"() -> (w749:bool)
                n238 = case shown="True" w749 {
                  frame False {
                    n239 = local read "Stopper that ends \nthe main loops"() -> (w751:bool)
                    n240 = local read "Start the Process"() -> (w750:bool)
                    n241 = Or(x=w751, y=w750) -> (x .or. y?=w752:bool)
                    n242 = case shown="False" w752 {
                      frame False {
                        n243 = while {
                          stop <- w755 stop-if-true
                          n244 = local read "Stop for End of \nExperiment \nand Data Writing"() -> (w754:bool)
                          n245 = local read "Stopper that ends \nthe main loops"() -> (w757:bool)
                          n246 = local read "Start the Process"() -> (w756:bool)
                          n247 = Wait (ms)(milliseconds to wait=u32 10) -> ()  [unwired: 1 out]
                          n248 = Or(x=w757, y=w756) -> (x .or. y?=w755:bool)
                          n249 = local write "Stopper that ends \nthe main loops"(w754) -> ()
                        }
                        n250 = One Button Dialog(message="Please Select the Process and Press 'Start the Process' Button") -> ()  [unwired: 1 in, 1 out]
                      }
                      frame True {
                      }
                    }
                  }
                  frame True {
                    n251 = stacked-sequence {
                      frame #0 {
                        n252 = for {
                          N: 1 -> [_]
                          n253 = stacked-sequence {
                            frame #0 {
                              # "Switch to Port-3"
                              # "Port-3 of pump is connected to Sample"
                              n254 = local read "VISA Refnum in\nfor Pump"() -> (w762:refnum<visa-resource-name>)
                              n255 = local write "Pause Data Collection"(TRUE ("Pause Data Collection")) -> ()
                              n256 = call "PortChanger (SubVI).vi"("Port Number"="3", "VISA Refnum in"=w762) -> ()  [unwired: 10 in]
                            }
                            frame #1 {
                              n257 = local read "VISA Refnum in\nfor Pump"() -> (w763:refnum<visa-resource-name>)
                              n258 = call "ProcessCompletionWaiter (SubVI).vi"("VISA Refnum in"=w763) -> ()  [unwired: 11 in]
                            }
                            frame #2 {
                              n259 = local read "VISA Refnum in\nfor Pump"() -> (w768:refnum<visa-resource-name>)
                              n260 = local read "Volume of Syringe"() -> (w767:dbl)
                              n261 = call "RPickUp(SubVI).vi"("Volume to be picked up"=10.0, "Volume of Syringe"=w767, "Resolution of PickUP"=T2."Standard Pumping", "PickUp Flow Rate (ul/min)"=15.0, "VISA Refnum in"=w768) -> ()  [unwired: 6 in, 1 out]
                            }
                            frame #3 {
                              n262 = local read "Stopper that ends \nthe main loops"() -> (w769:bool)
                              n263 = local read "VISA Refnum in\nfor Pump"() -> (w770:refnum<visa-resource-name>)
                              n264 = case shown="True" w769 {
                                frame False {
                                }
                                frame True {
                                n265 = local read "VISA Refnum in\nfor Pump"() -> (w771:refnum<visa-resource-name>)
                                n266 = call "HardStopCurrentProcess (SubVI).vi"("VISA Refnum in"=w771) -> ()  [unwired: 11 in]
                                }
                              }
                              n267 = call "ProcessCompletionWaiter (SubVI).vi"("VISA Refnum in"=w770) -> ()  [unwired: 11 in]
                            }
                            frame #4 {
                              # "Switch to Port-1"
                              # "Port-1 of the pump is conncted to Waste"
                              n268 = local read "VISA Refnum in\nfor Pump"() -> (w773:refnum<visa-resource-name>)
                              n269 = call "PortChanger (SubVI).vi"("Port Number"="1", "VISA Refnum in"=w773) -> ()  [unwired: 10 in]
                            }
                            frame #5 {
                              n270 = local read "Stopper that ends \nthe main loops"() -> (w774:bool)
                              n271 = local read "VISA Refnum in\nfor Pump"() -> (w775:refnum<visa-resource-name>)
                              n272 = case shown="True" w774 {
                                frame False {
                                }
                                frame True {
                                n273 = local read "VISA Refnum in\nfor Pump"() -> (w776:refnum<visa-resource-name>)
                                n274 = call "HardStopCurrentProcess (SubVI).vi"("VISA Refnum in"=w776) -> ()  [unwired: 11 in]
                                }
                              }
                              n275 = call "ProcessCompletionWaiter (SubVI).vi"("VISA Refnum in"=w775) -> ()  [unwired: 11 in]
                            }
                            frame #6 {
                              n276 = local read "VISA Refnum in\nfor Pump"() -> (w781:refnum<visa-resource-name>)
                              n277 = local read "Volume of Syringe"() -> (w780:dbl)
                              n278 = call "GoToAbsolutePosition(SubVI).vi"("Absolute Volume Position in Syringe (in ul)"=0.0 ("Volume to be Dispensed"), "Volume of Syringe"=w780, "Resolution of Pumping"=T2."Standard Pumping" ("Resolution for Dispensing"), "Flow Rate (ul/min)"=150.0 ("Dispense Flow Rate (ul/min)"), "VISA Refnum in"=w781) -> ()  [unwired: 6 in, 1 out]
                            }
                            frame #7 {
                              n279 = local read "Stopper that ends \nthe main loops"() -> (w783:bool)
                              n280 = case shown="True" w783 {
                                frame False {
                                }
                                frame True {
                                n281 = local read "VISA Refnum in\nfor Pump"() -> (w784:refnum<visa-resource-name>)
                                n282 = call "HardStopCurrentProcess (SubVI).vi"("VISA Refnum in"=w784) -> ()  [unwired: 11 in]
                                }
                              }
                              n283 = local read "VISA Refnum in\nfor Pump"() -> (w782:refnum<visa-resource-name>)
                              n284 = call "ProcessCompletionWaiter (SubVI).vi"("VISA Refnum in"=w782) -> ()  [unwired: 11 in]
                            }
                          }
                        }
                      }
                      frame #1 {
                        n285 = local write "Start the Process"(FALSE ("Start the Process")) -> ()
                      }
                    }
                  }
                }
              }
              frame True {
                n286 = local write "Pause Data Collection"(FALSE ("Pause Data Collection")) -> ()
              }
            }
          }
          frame "Clean the tubing from Port-<n> Vial" {
            n287 = local read "Stopper that ends \nthe main loops"() -> (w787:bool)
            n288 = case shown="False" w787 {
              frame False {
                n289 = local read "Start the Process"() -> (w788:bool)
                n290 = case shown="True" w788 {
                  frame False {
                    n291 = local read "Stopper that ends \nthe main loops"() -> (w790:bool)
                    n292 = local read "Start the Process"() -> (w789:bool)
                    n293 = Or(x=w790, y=w789) -> (x .or. y?=w791:bool)
                    n294 = case shown="False" w791 {
                      frame False {
                        n295 = while {
                          stop <- w794 stop-if-true
                          n296 = local read "Stopper that ends \nthe main loops"() -> (w796:bool)
                          n297 = local read "Stop for End of \nExperiment \nand Data Writing"() -> (w793:bool)
                          n298 = local read "Start the Process"() -> (w795:bool)
                          n299 = Wait (ms)(milliseconds to wait=u32 10) -> ()  [unwired: 1 out]
                          n300 = Or(x=w796, y=w795) -> (x .or. y?=w794:bool)
                          n301 = local write "Stopper that ends \nthe main loops"(w793) -> ()
                        }
                        n302 = One Button Dialog(message="Please Select the Process and Press 'Start the Process' Button") -> ()  [unwired: 1 in, 1 out]
                      }
                      frame True {
                      }
                    }
                  }
                  frame True {
                    n303 = stacked-sequence {
                      frame #0 {
                        n304 = local read "No. of \ncleaning cycles"() -> (w798:i32)
                        n305 = for {
                          N: w798 -> [_]
                          n306 = stacked-sequence {
                            frame #0 {
                              # "Switch to Port-4"
                              # "Port-4 of pump is connected to Buffer-A"
                              n307 = local read "VISA Refnum in\nfor Pump"() -> (w801:refnum<visa-resource-name>)
                              n308 = property on="Port-<n> to be \nCleaned (4-9)" class="Ring (strict)"() -> ("RingText.Text"=w799:string)  [unwired: 2 in, 2 out]
                              n309 = local write "Pause Data Collection"(TRUE ("Pause Data Collection")) -> ()
                              n310 = call "PortChanger (SubVI).vi"("Port Number"=w799, "VISA Refnum in"=w801) -> ()  [unwired: 10 in]
                            }
                            frame #1 {
                              n311 = local read "VISA Refnum in\nfor Pump"() -> (w802:refnum<visa-resource-name>)
                              n312 = call "ProcessCompletionWaiter (SubVI).vi"("VISA Refnum in"=w802) -> ()  [unwired: 11 in]
                            }
                            frame #2 {
                              n313 = local read "VISA Refnum in\nfor Pump"() -> (w807:refnum<visa-resource-name>)
                              n314 = local read "Apparent Volume\nof Syringe"() -> (w803:dbl)
                              n315 = local read "Volume of Syringe"() -> (w806:dbl)
                              n316 = call "RPickUp(SubVI).vi"("Volume to be picked up"=w803, "Volume of Syringe"=w806, "Resolution of PickUP"=T2."Standard Pumping", "PickUp Flow Rate (ul/min)"=150.0, "VISA Refnum in"=w807) -> ()  [unwired: 6 in, 1 out]
                            }
                            frame #3 {
                              n317 = local read "Stopper that ends \nthe main loops"() -> (w808:bool)
                              n318 = local read "VISA Refnum in\nfor Pump"() -> (w809:refnum<visa-resource-name>)
                              n319 = case shown="True" w808 {
                                frame False {
                                }
                                frame True {
                                n320 = local read "VISA Refnum in\nfor Pump"() -> (w810:refnum<visa-resource-name>)
                                n321 = call "HardStopCurrentProcess (SubVI).vi"("VISA Refnum in"=w810) -> ()  [unwired: 11 in]
                                }
                              }
                              n322 = call "ProcessCompletionWaiter (SubVI).vi"("VISA Refnum in"=w809) -> ()  [unwired: 11 in]
                            }
                            frame #4 {
                              # "Switch to Port-1"
                              # "Port-1 of the pump is conncted to Waste"
                              n323 = local read "VISA Refnum in\nfor Pump"() -> (w812:refnum<visa-resource-name>)
                              n324 = call "PortChanger (SubVI).vi"("Port Number"="1", "VISA Refnum in"=w812) -> ()  [unwired: 10 in]
                            }
                            frame #5 {
                              n325 = local read "Stopper that ends \nthe main loops"() -> (w813:bool)
                              n326 = local read "VISA Refnum in\nfor Pump"() -> (w814:refnum<visa-resource-name>)
                              n327 = case shown="True" w813 {
                                frame False {
                                }
                                frame True {
                                n328 = local read "VISA Refnum in\nfor Pump"() -> (w815:refnum<visa-resource-name>)
                                n329 = call "HardStopCurrentProcess (SubVI).vi"("VISA Refnum in"=w815) -> ()  [unwired: 11 in]
                                }
                              }
                              n330 = call "ProcessCompletionWaiter (SubVI).vi"("VISA Refnum in"=w814) -> ()  [unwired: 11 in]
                            }
                            frame #6 {
                              n331 = local read "VISA Refnum in\nfor Pump"() -> (w820:refnum<visa-resource-name>)
                              n332 = local read "Volume of Syringe"() -> (w819:dbl)
                              n333 = call "GoToAbsolutePosition(SubVI).vi"("Absolute Volume Position in Syringe (in ul)"=0.0 ("Volume to be Dispensed"), "Volume of Syringe"=w819, "Resolution of Pumping"=T2."Standard Pumping" ("Resolution for Dispensing"), "Flow Rate (ul/min)"=150.0 ("Dispense Flow Rate (ul/min)"), "VISA Refnum in"=w820) -> ()  [unwired: 6 in, 1 out]
                            }
                            frame #7 {
                              n334 = local read "Stopper that ends \nthe main loops"() -> (w822:bool)
                              n335 = case shown="True" w822 {
                                frame False {
                                }
                                frame True {
